vi "setStages.vi"(8 "error in (no error)":errorcluster, 10 "Stage":string, 11 "SingleToneRamp.lvclass in":refnum<class "SingleToneRamp.lvclass">) -> (0 "error out":errorcluster, 3 "SingleToneRamp.lvclass out":refnum<class "SingleToneRamp.lvclass">)   [LabVIEW 2011, in "Tools.lvlib" / "Scripting.lvlib" / "SingleToneRamp.lvclass"]
uses:
  SingleToneRamp.lvclass
  SingleTone.lvclass
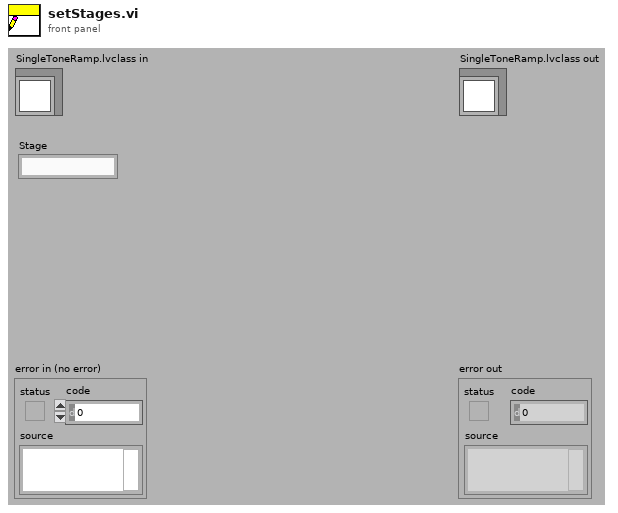
[diagram p1: front panel]
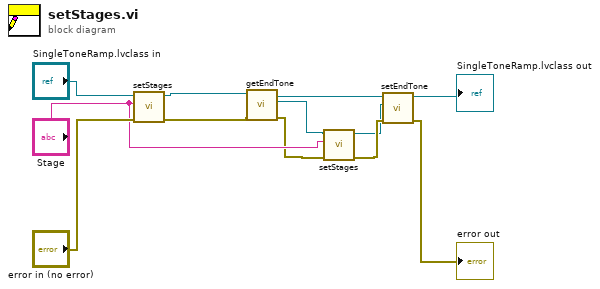
[diagram p0: block diagram]
diagram:
  n1 = call-parent "setStages.vi"("error in (no error)"="error in (no error)", "Stage"="Stage", "ScriptEvent.lvclass in"="SingleToneRamp.lvclass in") -> ("error out"=w7:errorcluster, "ScriptEvent.lvclass out"=w9:refnum<class "SingleToneRamp.lvclass">)  [unwired: 7 in]
  n2 = call "getEndTone.vi"("error in (no error)"=w7, "SingleToneRamp.lvclass in"=w9) -> ("error out"=w1:errorcluster, "endTone"=w3:refnum<class "SingleTone.lvclass">, "SingleToneRamp.lvclass out"=w10:refnum<class "SingleToneRamp.lvclass">)  [unwired: 7 in]
  n3 = call-dynamic "setStages.vi"("error in (no error)"=w1, "Stage"="Stage", "ScriptEvent.lvclass in"=w3) -> ("error out"=w5:errorcluster, "ScriptEvent.lvclass out"=w4:refnum<class "SingleTone.lvclass">)  [unwired: 7 in]
  n4 = call "setEndTone.vi"("error in (no error)"=w5, "EndTone"=w4, "SingleToneRamp.lvclass in"=w10) -> ("error out"=→"error out":errorcluster, "SingleToneRamp.lvclass out"=→"SingleToneRamp.lvclass out":refnum<class "SingleToneRamp.lvclass">)  [unwired: 7 in]
